vi "subSetSourcePathForExternalDeps.vi"(8 "error in (no error)":errorcluster, 9 "Dependency libs":T1, 11 "SolutionBuilder in":refnum<class "SolutionBuilder.lvclass">) -> (0 "error out":errorcluster, 3 "SolutionBuilder out":refnum<class "SolutionBuilder.lvclass">)   [LabVIEW 2020, in "SolutionBuilder.lvlib" / "SolutionBuilder.lvclass"]
uses:
  SolutionBuilder.lvclass
  Community/NamePathMap.ctl
  SolutionBuilder.lvclass/SolutionBuilder.ctl
  ProjectItem/ProjectItem.lvclass
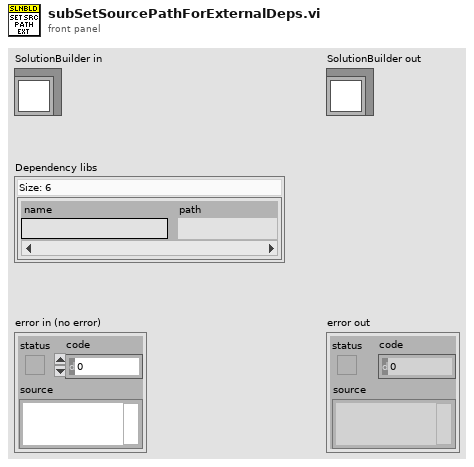
[diagram p1: front panel]
types:
  T1 = typedef "SolutionBuilder.lvlib/SolutionBuilder.lvclass/NamePathMap.ctl" = map{string, path}
  T2 = typedef "SolutionBuilder.lvlib/SolutionBuilder.lvclass/ProjectItemMap.ctl" = map{path, refnum<class "ProjectItem.lvclass">[]}
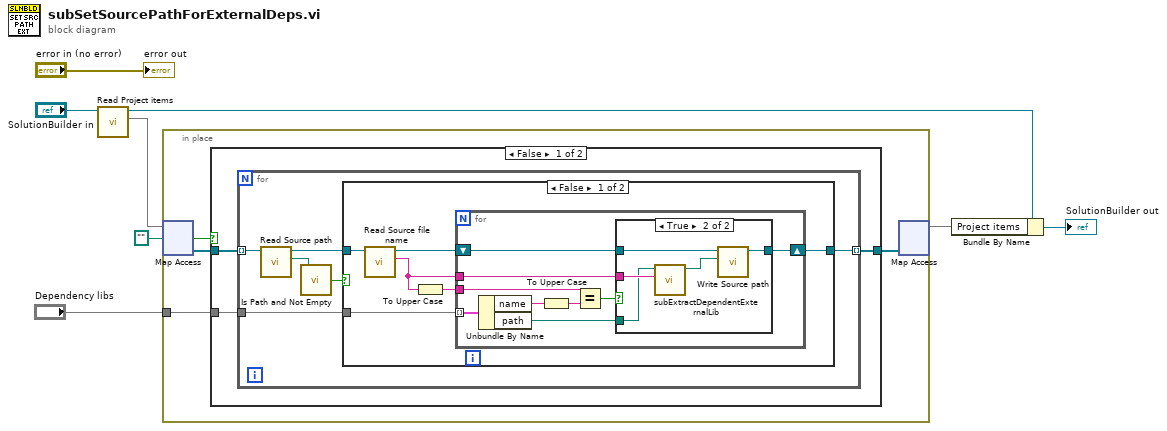
[diagram p0: block diagram]
diagram:
  n1 = call-dynamic "Read Project items.vi"("SolutionBuilder in"="SolutionBuilder in") -> ("Project items"=w2:T2, "SolutionBuilder out"=w7:refnum<class "SolutionBuilder.lvclass">)  [unwired: 9 in]
  n2 = in-place {
    in-place-border: "Dependency libs" -> [w9]
    n3 = in-place-map #1(w2, path "") -> (w10:refnum<class "ProjectItem.lvclass">[], w12:bool)  [unwired: 1 in]
    n4 = case shown="False" w12 {
      tunnel: [w13 w44] -> w11
      tunnel: w10 -> [w15 w44]
      tunnel: w9 -> [w14 _]
      frame False {
        n5 = for {
          tunnel: w15 -> [w18] mode=indexing
          tunnel: w14 -> [w21]
          tunnel: [w20] -> w13 mode=indexing
          n6 = call-dynamic "Read Source path.vi"("ProjectItem in"=w18) -> ("Source path"=w17:path, "ProjectItem out"=w19:refnum<class "ProjectItem.lvclass">)  [unwired: 9 in]
          n7 = call <vilib>:"Is Path and Not Empty.vi"("path"=w17) -> ("Is Path and Not Empty?"=w16:bool)  [unwired: 4 in]
          n8 = case shown="False" w16 {
            tunnel: w21 -> [w27 _]
            tunnel: [w24 w43] -> w20
            tunnel: w19 -> [w23 w43]
            frame False {
              n9 = call-dynamic "Read Source file name.vi"("ProjectItem in"=w23) -> ("Source file name"=w22:string, "ProjectItem out"=w25:refnum<class "ProjectItem.lvclass">)  [unwired: 9 in]
              n10 = To Upper Case(1:w22) -> (0:w26:string)
              n11 = for {
                tunnel: w27 -> [w36] mode=indexing
                tunnel: w26 -> [w29]
                shift-right: [w30] -> w24
                shift-left: w25 -> [w31]
                tunnel: w22 -> [w28]
                n12 = Unbundle By Name(w36) -> ("name"=w32:string, "path"=w33:path)
                n13 = To Upper Case(1:w32) -> (0:w35:string)
                n14 = Equal?(x=w29, y=w35) -> (x = y?=w34:bool)
                n15 = case shown="True" w34 {
                  tunnel: w33 -> [_ w38]
                  tunnel: w31 -> [w37 w42]
                  tunnel: [w37 w41] -> w30
                  tunnel: w28 -> [_ w40]
                  frame False {
                  }
                  frame True {
                    n16 = call "subExtractDependentExternalLib.vi"("Owning lib name"=w40, "Path"=w38) -> ("External lib"=w39:path)  [unwired: 9 in]
                    n17 = call-dynamic "Write Source path.vi"("Source path"=w39, "ProjectItem in"=w42) -> ("ProjectItem out"=w41:refnum<class "ProjectItem.lvclass">)  [unwired: 9 in]
                  }
                }
              }
            }
            frame True {
            }
          }
        }
      }
      frame True {
      }
    }
    n18 = in-place-map #1(w11) -> (w5:T2)  [unwired: 1 in, 2 out]
  }
  n19 = Bundle By Name(cluster=w7, "Project items"=w5) -> (→"SolutionBuilder out":refnum<class "SolutionBuilder.lvclass">)
  "error out" <- "error in (no error)"
